vi "UDP Data Share Receiver.vi"(6 "timeout ms (25000)":i32=1000, 8 "error in (no error)":errorcluster, 10 "max bytes/read":i32=548, 11 "Port":u16=61557) -> (0 "error out":errorcluster, 2 "Data Received":string)   [LabVIEW 2011]
doc: "This VI will read a single packet from the UDP port specified on the local host. This VI is meant to be used in a system where a VI is providing data to a web service. This VI will be run on the Web Service. The web service uses this VI to read data from the other running LabVIEW application. This is a replacement for shared variables, streams, TCP comm VIs, etc.\n\n\nVersion 1.0 - 02/13/2013\n\nPhaeron, Inc.\nwww.phaeron.com\ninfo@phaeron.com"
panel:
  out "# of Bytes Received":i32
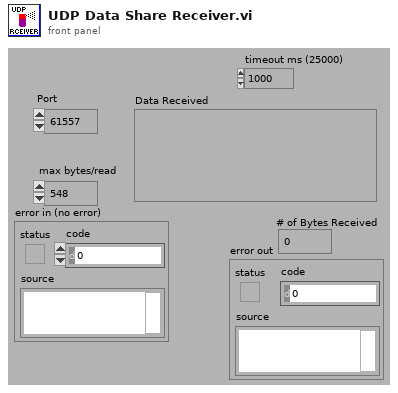
[diagram p1: front panel]
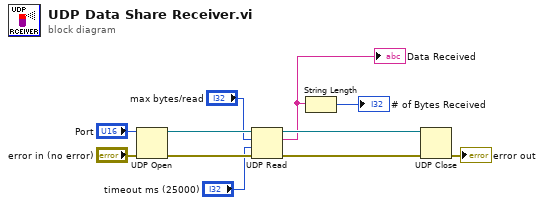
[diagram p0: block diagram]
diagram:
  n1 = UDP Open(8:"error in (no error)", 11:"Port") -> (port=w9:refnum<k16>, 0:w10:errorcluster)  [unwired: 3 in, 1 out]
  n2 = UDP Read(connection ID=w9, max size (548)="max bytes/read", timeout ms (25000)="timeout ms (25000)", 8:w10) -> (data out=w6:string, error out=w3:errorcluster, 3:w8:refnum<k16>)  [unwired: 2 out]
  "Data Received" <- w6
  n3 = String Length(string=w6) -> (length=→"# of Bytes Received":i32)
  n4 = UDP Close(connection ID=w8, 8:w3) -> (error out=→"error out":errorcluster)  [unwired: 1 out]
